vi "Barcode分组.vi"(11 "BarcodeArray":string[](array[string]) caption="第一行") -> (0 "条码信息":string, 2 "SN":string, 3 "ResultArray":string[](array[string]))   [LabVIEW 2011]
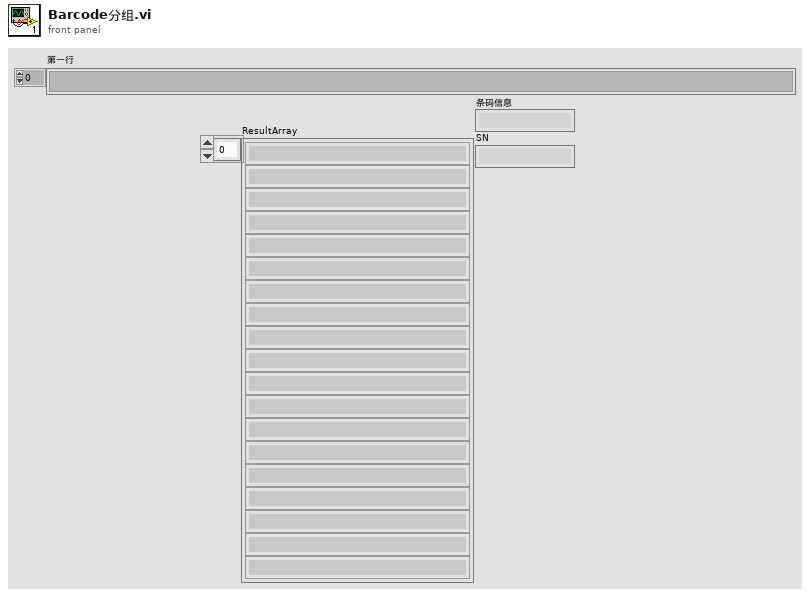
[diagram p1: front panel]
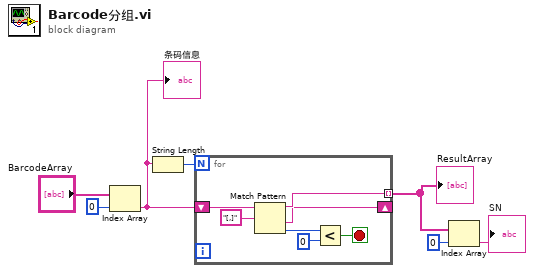
[diagram p0: block diagram]
diagram:
  n1 = Index Array(array="BarcodeArray", index=0 ("索引")) -> (element=w5:string)
  "条码信息" <- w5
  n2 = String Length(string=w5) -> (length=w4:i32)
  n3 = for {
    N: w4 -> [_]
    shift-right: [w9] -> _
    shift-left: w5 -> [w14]
    tunnel: [w10] -> w3 mode=indexing
    stop <- w8 stop-if-true
    n4 = Match Pattern(string=w14, regular expression="[,]" ("正则表达式")) -> (before substring=w10:string, after substring=w9:string, offset past match=w12:i32)  [unwired: 1 in, 1 out]
    n5 = Less?(x=w12, y=0) -> (x < y?=w8:bool)
  }
  "ResultArray" <- w3
  n6 = Index Array(array=w3, index=0 ("索引")) -> (element=→"SN":string)
